vi "WriteStringSpectrumAttribute.vi"() -> ()   [LabVIEW 2014, in "examples.lvlib"]
uses:
  examples.lvlib
  vis/tango_vi.llb/_TangoReadStringSpectrumAttribute.vi
  vis/tango_vi.llb/tango.lvlib
panel:
  out "x = y?":bool
  out "value":string[](array[string])
  out "write error out":errorcluster
  in  "write attribute name":string="string_spectrum_ro"
  in  "read-attribute name":string="string_spectrum_ro"
  in  "device name":string="sys/tg_test/1"
  out "?":string[](array[string])
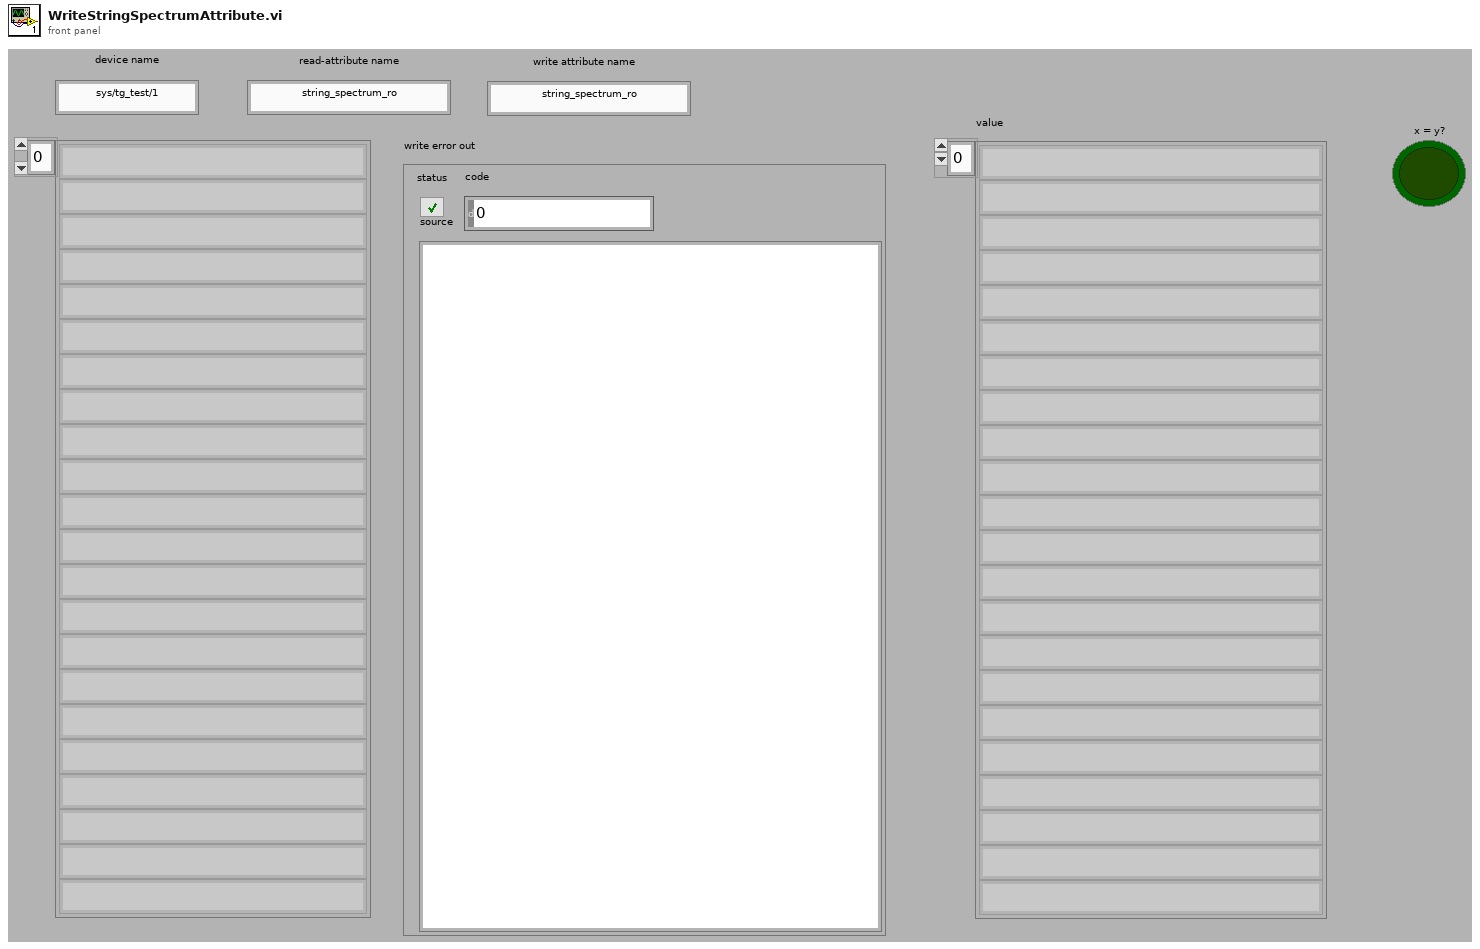
[diagram p1: front panel]
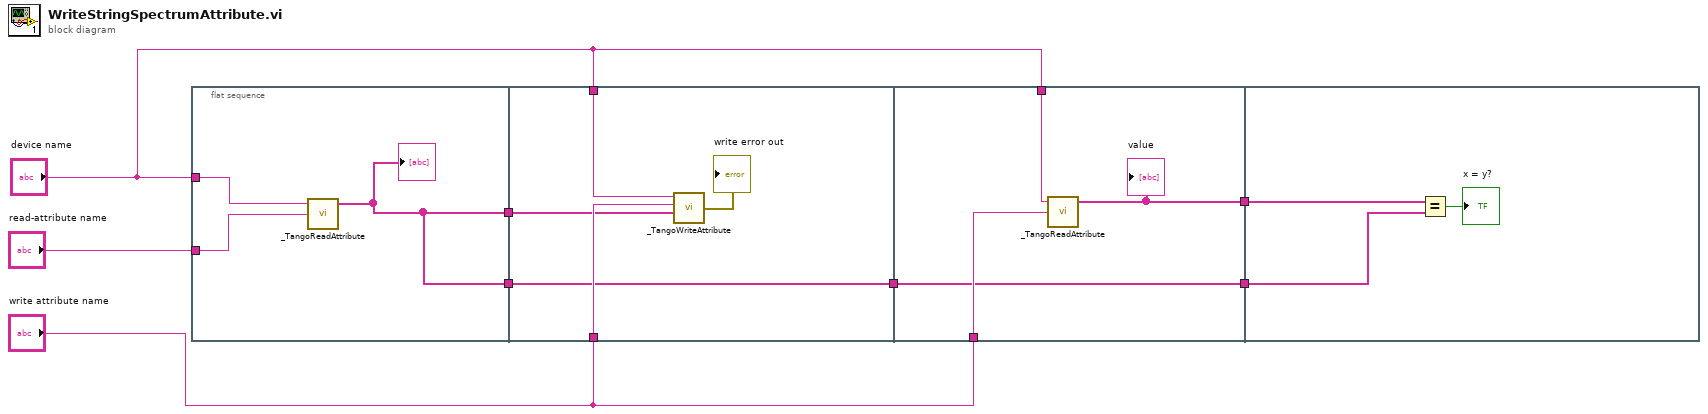
[diagram p0: block diagram]
diagram:
  n1 = flat-sequence {
    tunnel: "read-attribute name" -> [w11]
    tunnel: "device name" -> [w10]
    tunnel: [w9] -> w5
    tunnel: [w9] -> w1
    tunnel: "write attribute name" -> [w16]
    tunnel: "device name" -> [w15]
    tunnel: w5 -> [w13]
    tunnel: [w12] -> w2
    tunnel: w1 -> [w12]
    tunnel: "device name" -> [w20]
    tunnel: "write attribute name" -> [w19]
    tunnel: [w18] -> w4
    tunnel: [w17] -> w3
    tunnel: w2 -> [w17]
    tunnel: w4 -> [w23]
    tunnel: w3 -> [w22]
    frame #0 {
      n2 = call-poly "_TangoReadAttribute.vi"("attribute name"=w11, "device name"=w10) -> ("value"=w9:string[])  [unwired: 1 in, 2 out]
      "?" <- w9
    }
    frame #1 {
      n3 = call-poly "_TangoWriteAttribute.vi"("value"=w13, "attribute name"=w16, "device name"=w15) -> ("error out"=→"write error out":errorcluster)  [unwired: 1 in]
    }
    frame #2 {
      n4 = call-poly "_TangoReadAttribute.vi"("attribute name"=w19, "device name"=w20) -> ("value"=w18:string[])  [unwired: 1 in, 2 out]
      "value" <- w18
    }
    frame #3 {
      n5 = Equal?(x=w23, y=w22) -> (x = y?=→"x = y?":bool)
    }
  }
